vi "PRL Raw Data Viewer.vi"(9 "Raw Data":T1, 10 "Raw Data Channel Names":T2, 11 "Initialize":bool) -> ()   [LabVIEW 2013, in "PMU Recorder Light.lvlib"]
uses:
  PMU Recorder Light.lvlib
panel:
  in  "Angle View?":bool=TRUE
  out "Time Stamp":timestamp format="%<%.3X %x>T"
  out "Digital Channels":i32(listbox)=-1
  out "Analog Channels":i32(listbox)=-1
  out "Phasor Channels":i32(listbox)=-1
  in  "Update Rate":u32(ring)=1000 items=["10 Hz"=100, "5 Hz"=200, "2 Hz"=500, "1 Hz"=1000, "0.5 Hz"=2000, "0.2 Hz"=5000, "0.1 Hz"=10000]
  # "Re/Im"
  # "Amp/Ang"
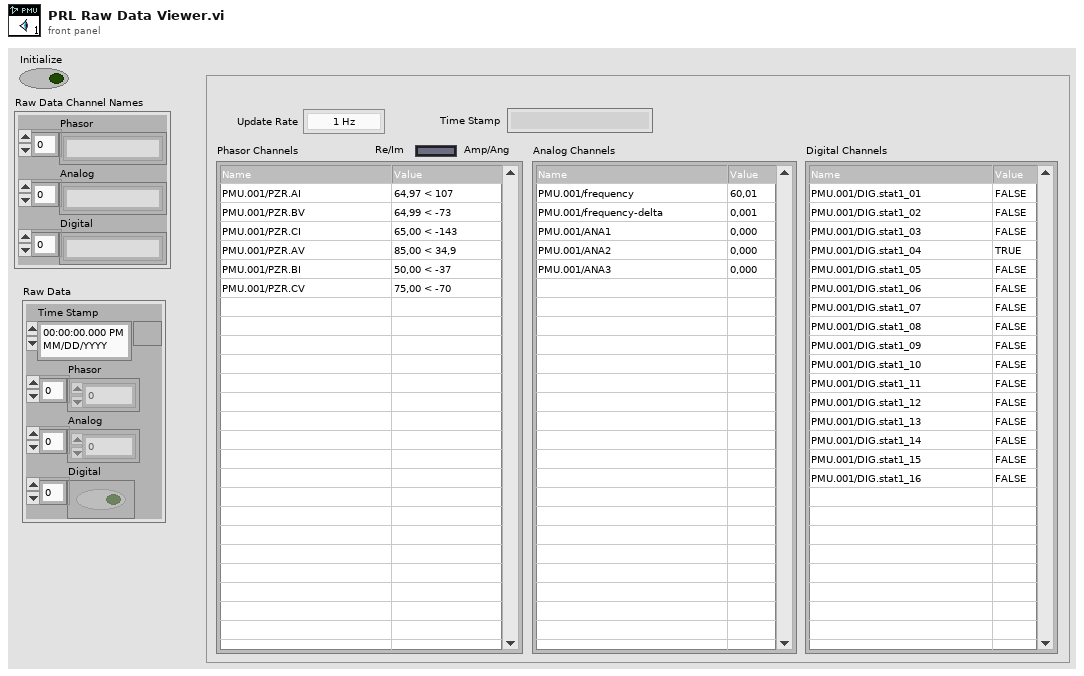
[diagram p1: front panel]
types:
  T1 = cluster{"Time Stamp":timestamp, "Phasor":csg[], "Analog":sgl[], "Digital":bool[]}
  T2 = cluster{"Phasor":string[], "Analog":string[], "Digital":string[]}
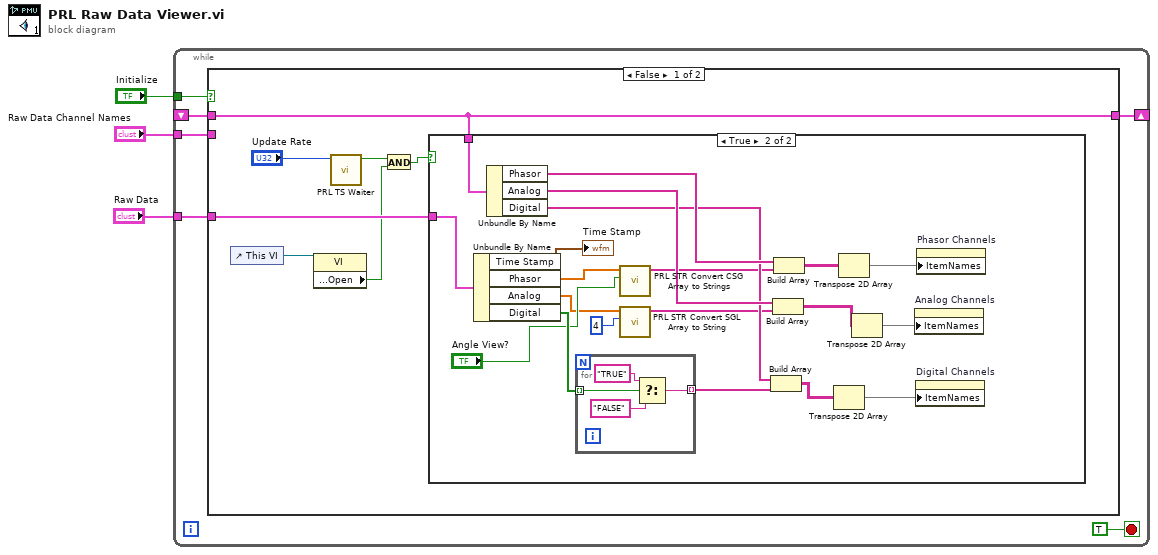
[diagram p0: block diagram]
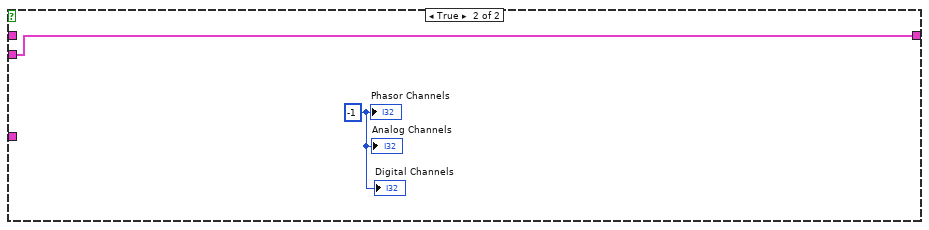
[diagram p3: hidden frame]
diagram:
  n1 = while {
    tunnel: "Initialize" -> [w8]
    shift-right: [w6] -> _
    shift-left: _ -> [w7]
    tunnel: "Raw Data Channel Names" -> [w5]
    tunnel: "Raw Data" -> [w4]
    stop <- TRUE stop-if-true
    n2 = case shown="False" w8 {
      tunnel: w7 -> [w16 _]
      tunnel: [w16 w42] -> w6
      tunnel: w5 -> [_ w42]
      tunnel: w4 -> [w15 _]
      frame False {
        n3 = control-ref of="This VI"() -> (w14:refnum<vi>)
        n4 = property class="VI"(reference=w14) -> ("Front Panel.Open"=w13:bool)  [unwired: 1 in, 2 out]
        n5 = call "PRL TS Waiter.vi"("Ms to Wait"="Update Rate") -> ("Trigger?"=w10:bool)  [unwired: 10 in]
        n6 = And(x=w10, y=w13) -> (x .and. y?=w12:bool)
        n7 = case shown="True" w12 {
          tunnel: w16 -> [_ w36]
          tunnel: w15 -> [_ w35]
          frame False {
          }
          frame True {
            n8 = Unbundle By Name(w35) -> ("Time Stamp"=→"Time Stamp":timestamp, "Phasor"=w21:csg[], "Analog"=w18:sgl[], "Digital"=w33:bool[])
            n9 = Unbundle By Name(w36) -> ("Phasor"=w32:string[], "Analog"=w31:string[], "Digital"=w29:string[])
            n10 = for {
              tunnel: w33 -> [w40] mode=indexing
              tunnel: [w37] -> w30 mode=indexing
              n11 = Select(t="TRUE" ("string"), s=w40, f="FALSE" ("string")) -> (s? t:f=w37:string)
            }
            n12 = call "PRL STR Convert CSG Array to Strings.vi"("Angle View?"="Angle View?", "Phasor"=w21) -> ("Strings"=w22:string[])  [unwired: 9 in]
            n13 = call "PRL STR Convert SGL Array to String.vi"("Precision"=4, "Values"=w18) -> ("Strings"=w19:string[])  [unwired: 9 in]
            n14 = Build Array(w29, w30) -> (w26:string[][])
            n15 = Build Array(w31, w19) -> (w27:string[][])
            n16 = Build Array(w32, w22) -> (w28:string[][])
            n17 = Transpose 2D Array(2D array=w26) -> (transposed array=w25:string[][])
            n18 = Transpose 2D Array(2D array=w28) -> (transposed array=w23:string[][])
            n19 = Transpose 2D Array(2D array=w27) -> (transposed array=w24:string[][])
            n20 = property on="Analog Channels" class="MCListbox (strict)"("ItemNames"=w24) -> ()  [unwired: 2 in, 2 out]
            n21 = property on="Digital Channels" class="MCListbox (strict)"("ItemNames"=w25) -> ()  [unwired: 2 in, 2 out]
            n22 = property on="Phasor Channels" class="MCListbox (strict)"("ItemNames"=w23) -> ()  [unwired: 2 in, 2 out]
          }
        }
      }
      frame True {
        w41 = -1 ("Phasor Channels")
        "Analog Channels" <- w41
        "Digital Channels" <- w41
        "Phasor Channels" <- w41
      }
    }
  }
